vi "Get StationGlobals.vi"(0 "Session Handle in":T2, 11 "error in (no error)":errorcluster) -> (4 "Session Handle out":T2, 8 "StationGlobals":T1, 15 "error out":errorcluster)   [LabVIEW 2020, in "TSS.lvlib" / "Engine.lvclass"]
uses:
  Engine/Engine.lvclass
  Engine/Typedefs/Session Handle.ctl
  Typedefs/Session Handle.ctl
  VariableContainer.lvclass
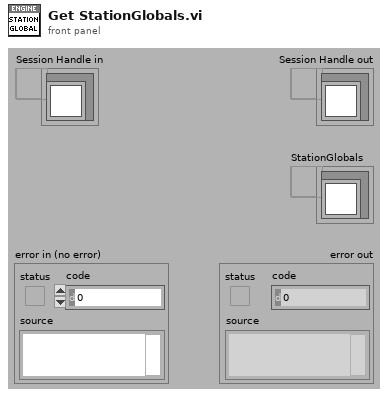
[diagram p1: front panel]
types:
  T1 = typedef "TSS.lvlib/VariableContainer.lvclass/Session Handle.ctl" = refnum<data-value>
  T2 = typedef "TSS.lvlib/Engine.lvclass/Session Handle.ctl" = refnum<data-value>
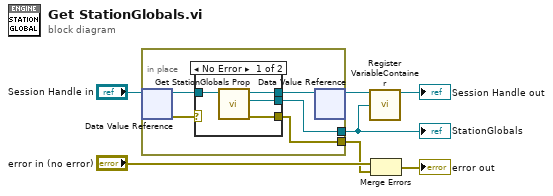
[diagram p0: block diagram]
diagram:
  n1 = in-place {
    in-place-border: [w9] -> w4
    in-place-border: [w8] -> w1
    n2 = in-place-dvr #1("Session Handle in") -> (w12:refnum<class "Engine.lvclass">, w10:errorcluster)
    n3 = case shown="No Error" w10 {
      selector: w10 -> [_ w18]
      tunnel: w12 -> [w16 w17]
      tunnel: [w15 w17] -> w11
      tunnel: [w14 w18] -> w9
      tunnel: [w13 _] -> w8
      frame No Error {
        n4 = call "Get StationGlobals Prop.vi"("TSEngine in"=w16) -> ("error out"=w14:errorcluster, "StationGlobals"=w13:T1, "TSEngine out"=w15:refnum<class "Engine.lvclass">)  [unwired: 8 in]
      }
      frame Error {
      }
    }
    n5 = in-place-dvr #1(w11) -> (w3:T2)  [unwired: 1 out]
  }
  "StationGlobals" <- w1
  n6 = call "Register VariableContainer.vi"("Engine  In"=w3, "VariableContainer"=w1) -> ("Engine"=→"Session Handle out":T2)  [unwired: 12 in, 1 out]
  n7 = Merge Errors("error in (no error)", w4) -> (→"error out":errorcluster)
